vi "CAM_ATTEMPT.vi"   [LabVIEW 2021]
uses:
  C:/Program Files/Thorlabs/Scientific Imaging/DCx Camera Support/Develop/DotNet/uc480DotNet.dll
  Program Files/Thorlabs/Scientific Imaging/DCx Camera Support/Develop/DotNet/uc480DotNet.dll
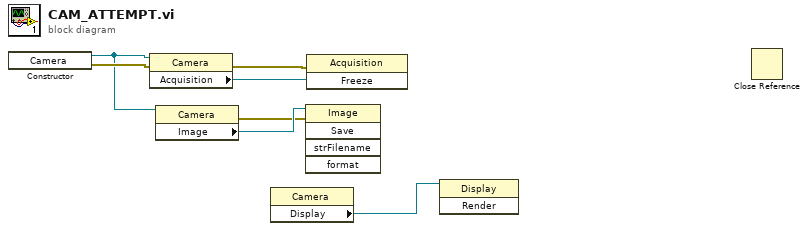
[diagram p0: block diagram]
diagram:
  n1 = constructor class="Camera"() -> (reference out=w3:refnum<k24>, error out=w5:errorcluster)  [unwired: 3 in, 1 out]
  n2 = property class="Camera"(reference=w3, error in=w5) -> (error out=w7:errorcluster, "Acquisition"=w6:refnum<k24>)  [unwired: 1 out]
  n3 = property class="Camera"(reference=w3) -> (error out=w1:errorcluster, "Image"=w2:refnum<k24>)  [unwired: 1 in, 1 out]
  n4 = property class="Camera"() -> ("Display"=w4:refnum<k24>)  [unwired: 2 in, 2 out]
  n5 = invoke class="Image" method="Save"(reference=w2, error in=w1) -> ()  [unwired: 3 in, 5 out]
  n6 = invoke class="Acquisition" method="Freeze"(reference=w6, error in=w7) -> ()  [unwired: 1 in, 3 out]
  n7 = invoke class="Display" method="Render"(reference=w4) -> ()  [unwired: 2 in, 3 out]
  n8 = Close Reference() -> ()  [unwired: 2 in, 1 out]
